vi "MungeInput.vi"(8 "error in (no error)":errorcluster, 10 "Input":string, 11 "BarCode in":refnum<class "BarCode.lvclass">) -> (0 "error out":errorcluster, 2 "Munged Input":string, 3 "BarCode out":refnum<class "BarCode.lvclass">)   [LabVIEW 2013, in "BarCodes.lvlib" / "BarCode.lvclass"]
doc: "Use this VI to modify the input to your barcode creating code. The munged input is passed to ValidateInput.vi, GetBars.vi, and WriteText.vi. The unchanged input is passed to WriteText.vi"
uses:
  BarCode.lvclass
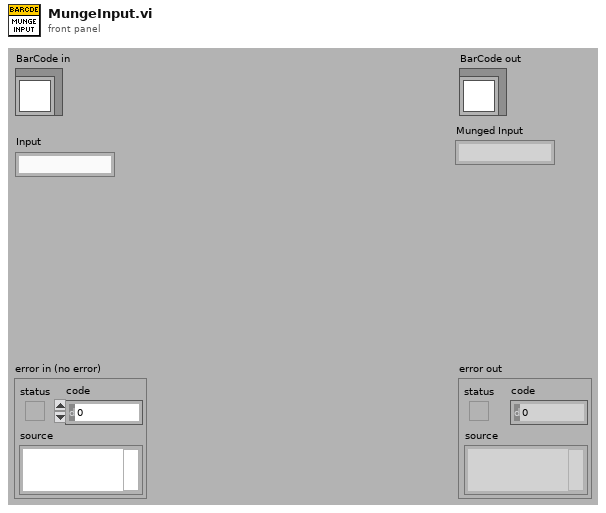
[diagram p1: front panel]
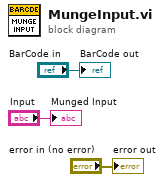
[diagram p0: block diagram]
diagram:
  "error out" <- "error in (no error)"
  "BarCode out" <- "BarCode in"
  "Munged Input" <- "Input"
